vi "LockDelta_RH_v2.vi"() -> ()   [LabVIEW 2019]
uses:
  <vilib>/Analysis/baseanly.llb/Mean (DBL).vi
  DeltaRamp_globals.vi
  B_Globals.vi
  Global 2.vi
  <vilib>/Analysis/NI_AALBase.lvlib
panel:
  out "Remote_Save_String":string
  in  "L1 ID":string
  in  "D1 ID":string="52A"
  out "read buffer":string
  out "R2":dbl=1.74102008
  in  "D1_use":bool=TRUE
  in  "L1_use":bool
  in  "D1":refnum<visa-resource-name>="GPIB1::20::INSTR"
  in  "L1":refnum<visa-resource-name>="GPIB1::7::INSTR"
  in  "Freq":dbl=71.34 format="%#_6e"
  out "B_set [T]":dbl
  in  "Reading Delay [ms]":i32=20 min=5
  in  "RW Delay":i32=5
  out "Exec Time [ms]":u32=29
  in  "B/T":bool=TRUE
  in  "Smart Avs":bool=TRUE
  in  "Points":dbl=1.0
  out "PpP":dbl=8.0
  in  "Combo Box":string(combo)="Temp"
  in  "Save":bool
  in  "Abort Delta":bool
  out "B [T]":dbl
  in  "Arm":bool
  in  "Measure":bool
  in  "I_Max":dbl=5e-05
  out "T":cluster{"X":dbl[], "Y":dbl[]}[](graph)=[{"X"=[300.2348517520214, 300.17, 300.17799999999994, 300.1689999999999, 300.166, 300.18, 300.186, 300.212, 300.20699999999994, 300.192, 300.183, 300.174, 300.167, 300.181, 300.1689999999999, 300.147, 300.157, 300.163, 300.166, 300.172, 300.184, 300.176, 300.16, 300.152, 300.16, 300.145, 300.12899999999996, 300.153, 300.157, 300.164, 300.153, 300.158, 300.154, 300.16800000000006, 300.184, 300.18800000000005, 300.176, 300.17900000000003, 300.1480000000001, 300.14899999999994, 300.15900000000005, 300.15799999999996, 300.147, 300.138, 300.135, 300.1360000000001, 300.162, 300.152, 300.146, 300.162, 300.167, 300.175, 300.16800000000006, 300.173, 300.189, 300.194, 300.183, 300.19700000000006, 300.19, 300.183, 300.15900000000005, 300.126, 300.12899999999996, 300.13900000000007, 300.12899999999996, 300.099, 300.048, 300.029, 299.998, 299.936, 299.74499999999995, 299.46599999999995, 299.114, 298.872, 298.507, 298.157, 297.859, 297.579, 297.412, 297.182, 297.0059999999999, 296.854, 296.76400000000007, 296.657, 296.56300000000005, 296.491, 296.433, 296.375, 296.334, 296.319, 296.305, 296.27, 296.262, 296.25500000000005, 296.263, 296.27399999999994, 296.29300000000006, 296.32099999999997, 296.347, 296.383, 296.4189999999999, 296.449, 296.502, 296.57099999999997, 296.673, 296.728, 296.81, 296.886, 296.987, 297.075, 297.157, 297.282, 297.405, 297.542, 297.69700000000006, 297.782, 297.923, 298.048, 298.181, 298.263, 298.39899999999994, 298.537, 298.67, 298.799, 298.88900000000007, 299.002, 299.125, 299.252, 299.34, 299.45, 299.58199999999994, 299.709, 299.809, 299.872, 299.968, 300.061, 300.147, 300.23500000000007, 300.288, 300.36999999999995, 300.449, 300.511, 300.564, 300.59999999999997, 300.65900000000005, 300.7060000000001, 300.753, 300.796, 300.819, 300.839, 300.867, 300.887, 300.92900000000003, 300.951, 300.961, 300.98500000000007, 300.992, 301.00399999999996, 301.01400000000007, 301.01, 301.019, 301.017, 301.012, 301.00399999999996, 300.991, 300.969, 300.959, 300.9560000000001, 300.954, 300.93, 300.925, 300.921, 300.913, 300.904, 300.88900000000007, 300.855, 300.846, 300.833, 300.825, 300.786, 300.788], "Y"=[nan, nan, nan, nan, nan, nan, nan, nan, nan, nan, nan, nan, nan, nan, nan, nan, nan, nan, nan, nan, nan, nan, nan, nan, nan, nan, nan, nan, nan, nan, nan, nan, nan, nan, nan, nan, nan, nan, nan, nan, nan, nan, nan, nan, nan, nan, nan, nan, nan, nan, nan, nan, nan, nan, nan, nan, nan, nan, nan, nan, nan, nan, nan, nan, nan, nan, nan, nan, nan, nan, nan, nan, nan, nan, nan, nan, nan, nan, nan, nan, nan, nan, nan, nan, nan, nan, nan, nan, nan, nan, nan, nan, nan, nan, nan, nan, nan, nan, nan, nan, nan, nan, nan, nan, nan, nan, nan, nan, nan, nan, nan, nan, nan, nan, nan, nan, nan, nan, nan, nan, nan, nan, nan, nan, nan, nan, nan, nan, nan, nan, nan, nan, nan, nan, nan, nan, nan, nan, nan, nan, nan, nan, nan, nan, nan, nan, nan, nan, nan, nan, nan, nan, nan, nan, nan, nan, nan, nan, nan, nan, nan, nan, nan, nan, nan, nan, nan, nan, nan, nan, nan, nan, nan, nan, nan, nan, nan, nan, nan, nan, nan]}, {"X"=[300.2348517520214, 300.17, 300.17799999999994, 300.1689999999999, 300.166, 300.18, 300.186, 300.212, 300.20699999999994, 300.192, 300.183, 300.174, 300.167, 300.181, 300.1689999999999, 300.147, 300.157, 300.163, 300.166, 300.172, 300.184, 300.176, 300.16, 300.152, 300.16, 300.145, 300.12899999999996, 300.153, 300.157, 300.164, 300.153, 300.158, 300.154, 300.16800000000006, 300.184, 300.18800000000005, 300.176, 300.17900000000003, 300.1480000000001, 300.14899999999994, 300.15900000000005, 300.15799999999996, 300.147, 300.138, 300.135, 300.1360000000001, 300.162, 300.152, 300.146, 300.162, 300.167, 300.175, 300.16800000000006, 300.173, 300.189, 300.194, 300.183, 300.19700000000006, 300.19, 300.183, 300.15900000000005, 300.126, 300.12899999999996, 300.13900000000007, 300.12899999999996, 300.099, 300.048, 300.029, 299.998, 299.936, 299.74499999999995, 299.46599999999995, 299.114, 298.872, 298.507, 298.157, 297.859, 297.579, 297.412, 297.182, 297.0059999999999, 296.854, 296.76400000000007, 296.657, 296.56300000000005, 296.491, 296.433, 296.375, 296.334, 296.319, 296.305, 296.27, 296.262, 296.25500000000005, 296.263, 296.27399999999994, 296.29300000000006, 296.32099999999997, 296.347, 296.383, 296.4189999999999, 296.449, 296.502, 296.57099999999997, 296.673, 296.728, 296.81, 296.886, 296.987, 297.075, 297.157, 297.282, 297.405, 297.542, 297.69700000000006, 297.782, 297.923, 298.048, 298.181, 298.263, 298.39899999999994, 298.537, 298.67, 298.799, 298.88900000000007, 299.002, 299.125, 299.252, 299.34, 299.45, 299.58199999999994, 299.709, 299.809, 299.872, 299.968, 300.061, 300.147, 300.23500000000007, 300.288, 300.36999999999995, 300.449, 300.511, 300.564, 300.59999999999997, 300.65900000000005, 300.7060000000001, 300.753, 300.796, 300.819, 300.839, 300.867, 300.887, 300.92900000000003, 300.951, 300.961, 300.98500000000007, 300.992, 301.00399999999996, 301.01400000000007, 301.01, 301.019, 301.017, 301.012, 301.00399999999996, 300.991, 300.969, 300.959, 300.9560000000001, 300.954, 300.93, 300.925, 300.921, 300.913, 300.904, 300.88900000000007, 300.855, 300.846, 300.833, 300.825, 300.786, 300.788], "Y"=[1.7447801286792448, 1.7447222037500003, 1.7444892225, 1.7447247049999999, 1.7444935777777777, 1.7447010424999998, 1.7444126299999998, 1.7446228562500001, 1.7444523166666668, 1.7446782055555554, 1.7442503550000001, 1.7445815471428572, 1.7445446699999998, 1.7444733666666667, 1.74438583625, 1.74470474, 1.74432511625, 1.7444609047058823, 1.7444559175000003, 1.74453283875, 1.74436205, 1.74448020875, 1.74424474, 1.74459511, 1.7443100344444444, 1.7445789274999999, 1.7443861512499996, 1.7446031822222219, 1.7441049224999998, 1.74444188, 1.74417156, 1.7444447835294117, 1.74440267625, 1.7443347725000002, 1.74462658125, 1.7443272925, 1.7443892799999998, 1.7444658800000001, 1.74426717875, 1.7445588900000002, 1.7442914700000003, 1.7443815285714288, 1.7442203222222221, 1.7444356812500001, 1.7443279187500003, 1.7443443888235295, 1.7443939437500002, 1.74418871125, 1.744245395, 1.74435906125, 1.7442560699999998, 1.744363755, 1.7442435012500002, 1.7443550225000002, 1.744275161111111, 1.7444952322222225, 1.7442897475000003, 1.7442084155555557, 1.74446526125, 1.744032623333333, 1.7444503137499998, 1.74405478, 1.7443459487499997, 1.7442460844444443, 1.7442503712500002, 1.74424321875, 1.7442301224999996, 1.7443053200000003, 1.7443908711111114, 1.7441522625, 1.7443821125, 1.7443603274999997, 1.74452349625, 1.7445079087499997, 1.7445287322222223, 1.74465774, 1.7443728855555556, 1.7443117199999998, 1.744500492222222, 1.7439781575, 1.74443067625, 1.7438763237500001, 1.7443025377777777, 1.7439469600000002, 1.7432400377777781, 1.74333129625, 1.7434138362499998, 1.7431936575000002, 1.7430730922222224, 1.7426461137499998, 1.7430441525, 1.7426726075, 1.7428233350000002, 1.74276167125, 1.74255301125, 1.74272678625, 1.7424671522222224, 1.74262526625, 1.74249634125, 1.7425897587499999, 1.742324008888889, 1.7426337, 1.7422789637499998, 1.7422661775, 1.742301568888889, 1.74232783875, 1.74205565625, 1.7423048024999999, 1.7421523744444443, 1.741956101111111, 1.7423072912499997, 1.74186632, 1.7423694011111113, 1.7417824999999998, 1.7421789288888891, 1.7418095787499999, 1.74209737875, 1.74203477625, 1.7418068633333332, 1.74197279, 1.74173145, 1.7420101762500002, 1.7416327388888888, 1.7419502722222222, 1.74192201875, 1.74173143625, 1.7418395262500002, 1.7417157888888888, 1.74199148875, 1.74175852625, 1.74190086125, 1.7415953755555555, 1.742182105, 1.7419347633333333, 1.74175076125, 1.741818508888889, 1.74180181375, 1.74189556875, 1.7418619544444445, 1.7418426124999997, 1.7420506762499999, 1.7416219577777778, 1.7419721533333334, 1.7416080975, 1.7417956928571425, 1.7416463144444445, 1.7418566212500002, 1.7418234744444443, 1.7418127074999998, 1.742116705, 1.7417476175000002, 1.7418373433333332, 1.74178592875, 1.7417111975, 1.7420812188888888, 1.7416140275, 1.742021707777778, 1.741713985, 1.74195474375, 1.7416716374999999, 1.7419106966666666, 1.741797445, 1.741861925, 1.7417786377777775, 1.7419472487500003, 1.7416695899999999, 1.74205845625, 1.7417355025, 1.742054368888889, 1.74172237625, 1.74197687, 1.7418625233333334, 1.74192047125, 1.7420078655555553, 1.74175012125, 1.7421686799999998, 1.74217179375, 1.74163177625, 1.741930425, 1.7418367466666664, 1.7420905387499999]}] caption="XY Graph"
  in  "Reset":bool
  out "Spl T [K]":dbl=300.783
  out "R1 [Ohm]":dbl=nan
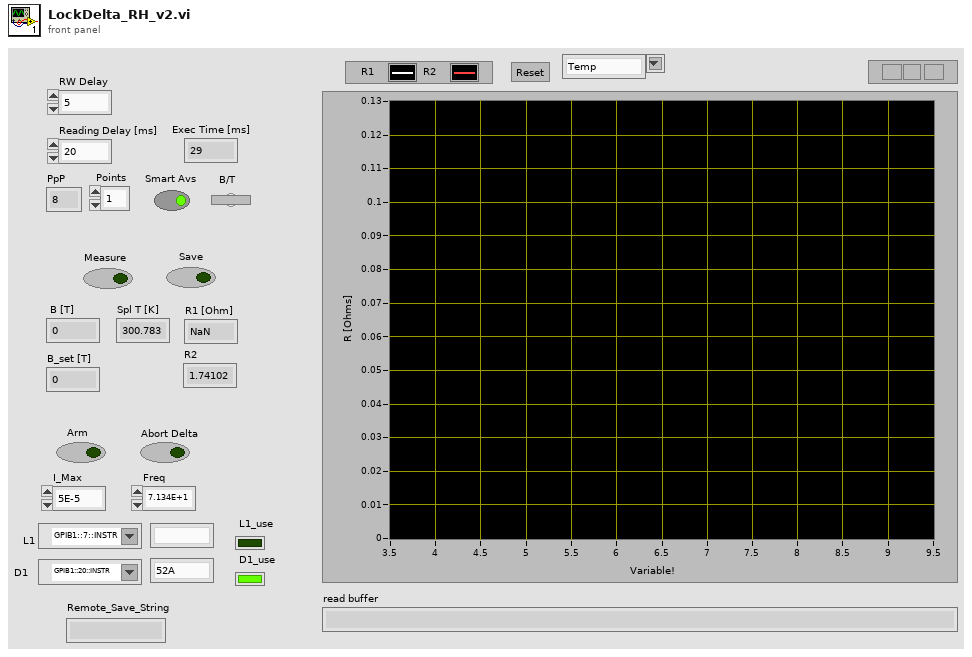
[diagram p1: front panel]
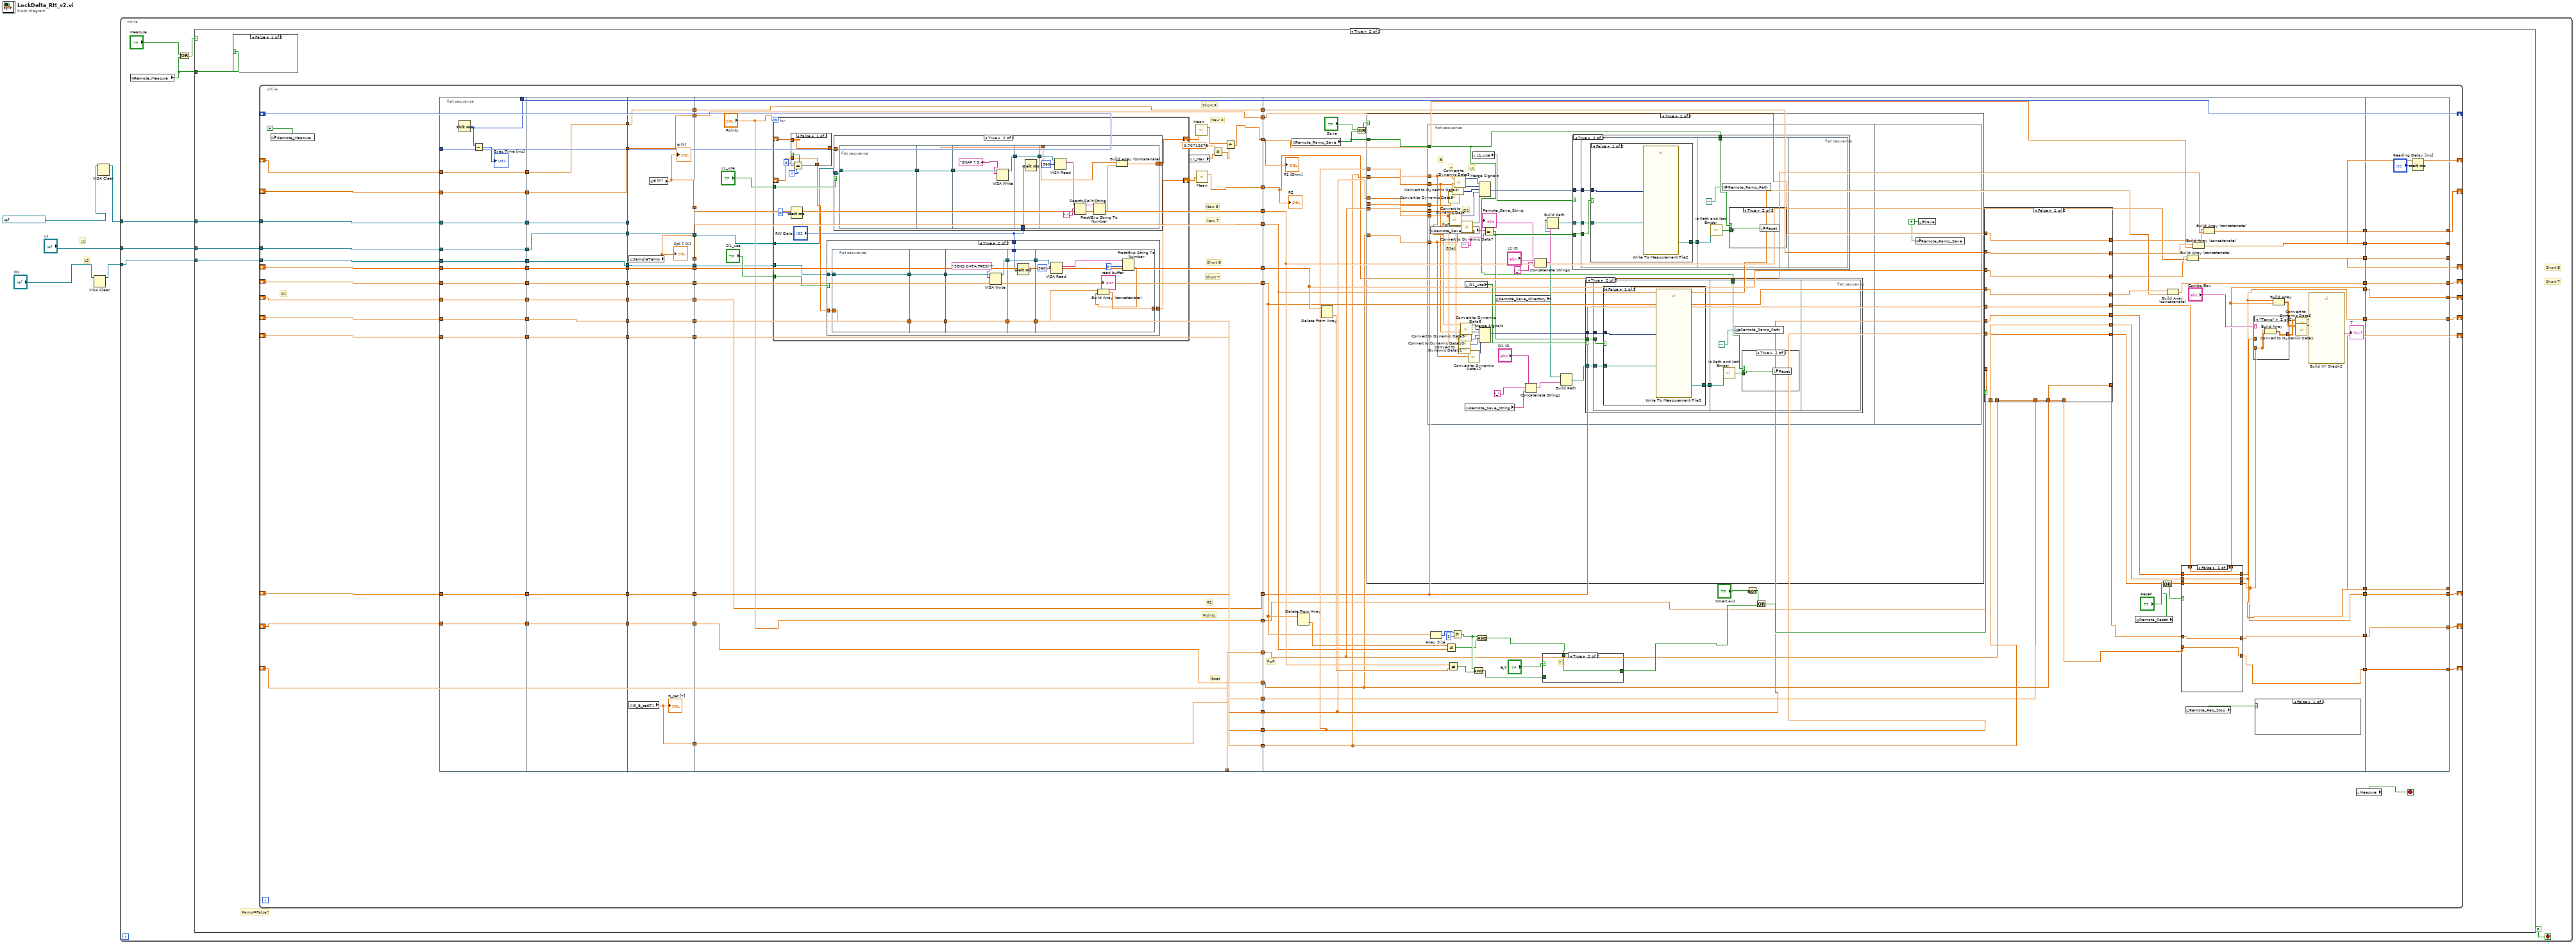
[diagram p0: block diagram]
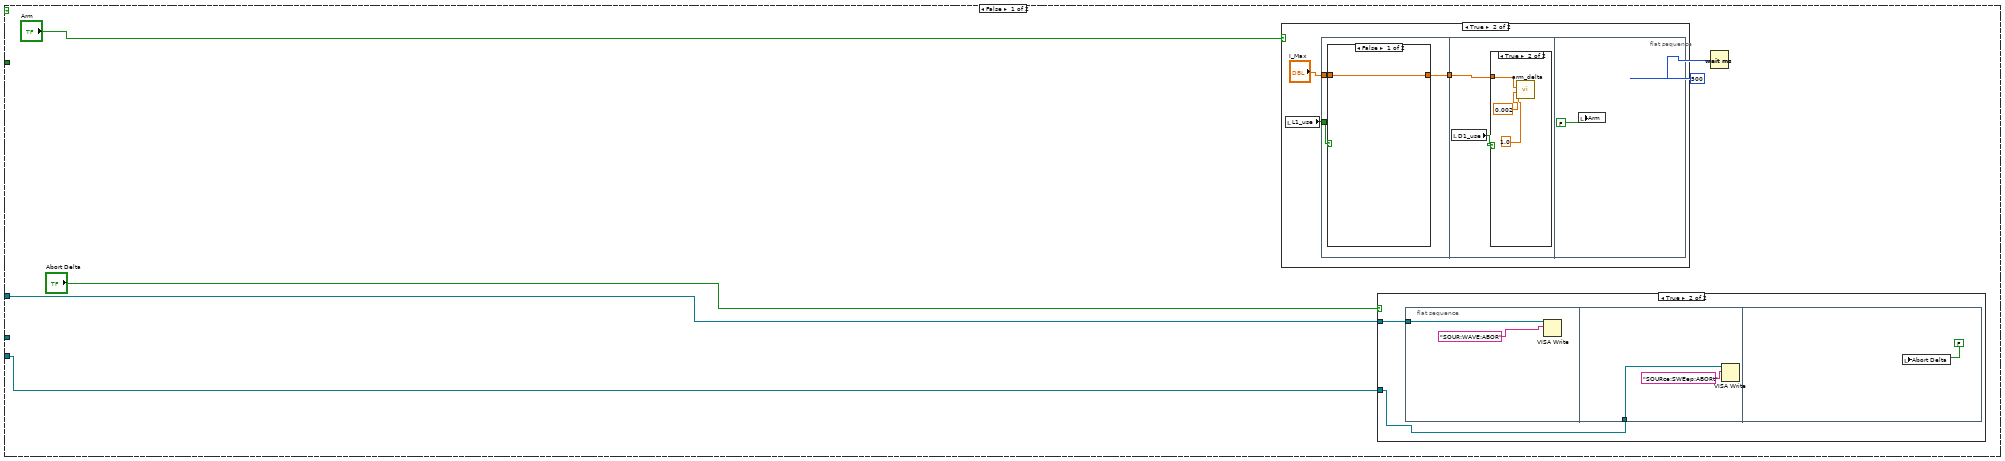
[diagram p2: hidden frame]
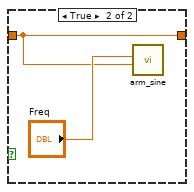
[diagram p5: hidden frame]
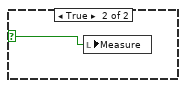
[diagram p7: hidden frame]
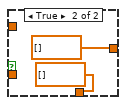
[diagram p10: hidden frame]
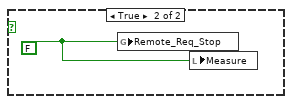
[diagram p12: hidden frame]
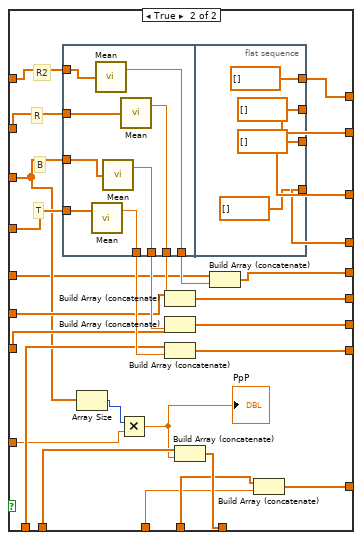
[diagram p13: hidden frame]
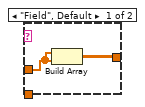
[diagram p14: hidden frame]
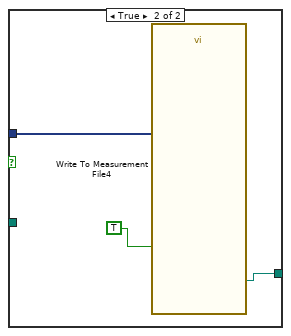
[diagram p17: hidden frame]
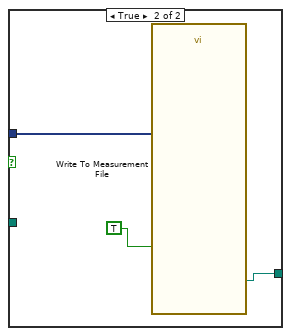
[diagram p20: hidden frame]
diagram:
  # "L2"
  # "L1"
  n1 = VISA Clear(VISA resource name="D1") -> (VISA resource name out=w1:refnum<visa-resource-name>)  [unwired: 1 in, 1 out]
  n2 = VISA Clear(VISA resource name=refnum<visa-resource-name> "GPIB1::22::INSTR" ("Keithley")) -> (VISA resource name out=w5:refnum<visa-resource-name>)  [unwired: 1 in, 1 out]
  n3 = while {
    tunnel: w5 -> [w11]
    tunnel: "L1" -> [w7]
    tunnel: w1 -> [w6]
    stop <- FALSE stop-if-true
    # "Short T"
    # "Short B"
    n4 = global read "DeltaRamp_globals.vi" "Remote_Measure"() -> (w8:bool)
    n5 = Or(x="Measure", y=w8) -> (x .or. y?=w10:bool)
    n6 = case shown="True" w10 {
      tunnel: w11 -> [w15 w43]
      tunnel: w8 -> [_ w42]
      tunnel: w7 -> [_ w41]
      tunnel: w6 -> [w13 w40]
      frame False {
        n7 = case shown="True" "Arm" {
          frame False {
          }
          frame True {
            n8 = local read "L1_use"() -> (w25:bool)
            n9 = flat-sequence {
              tunnel: [w30] -> w27
              tunnel: "I_Max" -> [w29]
              tunnel: w25 -> [w28]
              tunnel: w27 -> [w35]
              frame #0 {
                n10 = case shown="False" w28 {
                  tunnel: [w31 w32] -> w30
                  tunnel: w29 -> [w31 w32]
                  frame False {
                  }
                  frame True {
                    n11 = call "arm_sine.vi"("Peak Amp"=w32, "Freq"="Freq") -> ()  [unwired: 10 in]
                  }
                }
              }
              frame #1 {
                n12 = local read "D1_use"() -> (w34:bool)
                n13 = case shown="True" w34 {
                  tunnel: w35 -> [_ w38]
                  frame False {
                  }
                  frame True {
                    n14 = call "arm_delta.vi"("Compliance [V]"=1.0, "DELAY [sec]"=0.002, "I-HIGH [A]"=w38) -> ()  [unwired: 9 in]
                  }
                }
              }
              frame #2 {
                n15 = local write "Arm"(FALSE) -> ()
              }
            }
          }
        }
        n16 = case shown="True" "Abort Delta" {
          tunnel: w15 -> [_ w19]
          tunnel: w13 -> [_ w18]
          frame False {
          }
          frame True {
            n17 = flat-sequence {
              tunnel: w19 -> [w21]
              tunnel: w18 -> [w22]
              frame #0 {
                n18 = VISA Write(VISA resource name=w21, write buffer="SOUR:WAVE:ABOR") -> ()  [unwired: 1 in, 3 out]
              }
              frame #1 {
                n19 = VISA Write(VISA resource name=w22, write buffer="SOURce:SWEep:ABORt") -> ()  [unwired: 1 in, 3 out]
              }
              frame #2 {
                n20 = local write "Abort Delta"(FALSE) -> ()
              }
            }
          }
        }
        n21 = Wait (ms)(milliseconds to wait=500) -> ()  [unwired: 1 out]
      }
      frame True {
        # "Ramp=False?"
        n22 = case shown="False" w42 {
          selector: w42 -> [_ w44]
          frame False {
          }
          frame True {
            n23 = local write "Measure"(w44) -> ()
          }
        }
        n24 = while {
          shift-right: [w87] -> _
          shift-left: _ -> [w94]
          shift-right: [w106] -> _
          shift-left: _ -> [w111]
          tunnel: w43 -> [w129]
          shift-right: [w104] -> _
          shift-left: _ -> [w117]
          shift-right: [w86] -> _
          shift-left: _ -> [w98]
          shift-right: [w88] -> _
          shift-left: _ -> [w103]
          shift-right: [w105] -> _
          shift-left: _ -> [w121]
          shift-right: [w130] -> _
          shift-left: _ -> [w131]
          shift-right: [w133] -> _
          shift-left: _ -> [w134]
          shift-right: [w70] -> _
          shift-left: _ -> [w75]
          tunnel: w41 -> [w67]
          tunnel: w40 -> [w66]
          shift-right: [w52] -> _
          shift-left: _ -> [w57]
          shift-right: [w50] -> _
          shift-left: _ -> [w48]
          stop <- w77 stop-if-true
          # "R2"
          n25 = global write "DeltaRamp_globals.vi" "Remote_Measure"(FALSE) -> ()
          n26 = flat-sequence {
            tunnel: w134 -> [w150]
            tunnel: [w148] -> w133
            tunnel: w129 -> [w147]
            tunnel: [w147] -> w127
            tunnel: w121 -> [w146]
            tunnel: [w146] -> w120
            tunnel: w117 -> [w145]
            tunnel: [w145] -> w114
            tunnel: w111 -> [w144]
            tunnel: [w144] -> w109
            tunnel: w103 -> [w143]
            tunnel: [w143] -> w100
            tunnel: [w142] -> w99
            tunnel: w98 -> [w142]
            tunnel: [w141] -> w95
            tunnel: w94 -> [w141]
            tunnel: [w140] -> w76
            tunnel: w75 -> [w140]
            tunnel: w67 -> [w139]
            tunnel: w66 -> [w138]
            tunnel: [w139] -> w65
            tunnel: [w138] -> w64
            tunnel: [w137] -> w58
            tunnel: w57 -> [w137]
            tunnel: [w136] -> w49
            tunnel: w48 -> [w136]
            tunnel: [w162] -> w128
            tunnel: w127 -> [w162]
            tunnel: w120 -> [w161]
            tunnel: [w161] -> w119
            tunnel: [w160] -> w115
            tunnel: w114 -> [w160]
            tunnel: [w159] -> w110
            tunnel: w109 -> [w159]
            tunnel: [w158] -> w101
            tunnel: w100 -> [w158]
            tunnel: w99 -> [w157]
            tunnel: [w157] -> w96
            tunnel: w95 -> [w156]
            tunnel: [w156] -> w92
            tunnel: w76 -> [w155]
            tunnel: [w155] -> w73
            tunnel: w65 -> [w154]
            tunnel: w64 -> [w153]
            tunnel: [w154] -> w62
            tunnel: [w153] -> w60
            tunnel: w58 -> [w152]
            tunnel: [w152] -> w56
            tunnel: w49 -> [w151]
            tunnel: [w151] -> w46
            tunnel: w128 -> [_]
            tunnel: [w176] -> w125
            tunnel: [w175] -> w123
            tunnel: w119 -> [w174]
            tunnel: [w174] -> w118
            tunnel: [w173] -> w116
            tunnel: w115 -> [w173]
            tunnel: w110 -> [w172]
            tunnel: [w172] -> w108
            tunnel: [w171] -> w102
            tunnel: w101 -> [w171]
            tunnel: [w170] -> w97
            tunnel: w96 -> [w170]
            tunnel: [w169] -> w93
            tunnel: w92 -> [w169]
            tunnel: [w168] -> w74
            tunnel: w73 -> [w168]
            tunnel: [w167] -> w69
            tunnel: [w166] -> w63
            tunnel: w62 -> [w166]
            tunnel: [w165] -> w61
            tunnel: w60 -> [w165]
            tunnel: w56 -> [w164]
            tunnel: [w164] -> w54
            tunnel: [w163] -> w47
            tunnel: w46 -> [w163]
            tunnel: [w201] -> w132
            tunnel: w131 -> [w201]
            tunnel: [w181] -> w126
            tunnel: w125 -> [w200]
            tunnel: [w200] -> w124
            tunnel: w123 -> [w199]
            tunnel: [w199] -> w122
            tunnel: w118 -> [w198]
            tunnel: w116 -> [w197]
            tunnel: [w198] -> w113
            tunnel: [w197] -> w112
            tunnel: w108 -> [w196]
            tunnel: [w196] -> w107
            tunnel: w102 -> [w195]
            tunnel: w97 -> [w194]
            tunnel: w93 -> [w193]
            tunnel: [w195] -> w91
            tunnel: [w194] -> w90
            tunnel: [w193] -> w89
            tunnel: ["Points"] -> w85
            tunnel: w74 -> [w191]
            tunnel: [w191] -> w72
            tunnel: w69 -> [w190]
            tunnel: [w190] -> w68
            tunnel: w63 -> [w186]
            tunnel: w61 -> [w187]
            tunnel: [w177] -> w59
            tunnel: [w183] -> w55
            tunnel: w54 -> [w183]
            tunnel: w47 -> [w182]
            tunnel: [w182] -> w45
            tunnel: w132 -> [w313]
            tunnel: w126 -> [w305]
            tunnel: w124 -> [w304]
            tunnel: w122 -> [w300]
            tunnel: w113 -> [w309]
            tunnel: w112 -> [w303]
            tunnel: w107 -> [w308]
            tunnel: w91 -> [w292]
            tunnel: w90 -> [w291]
            tunnel: w89 -> [w290]
            tunnel: w85 -> [w296]
            tunnel: [w297] -> w84
            tunnel: [w306] -> w83
            tunnel: [w302] -> w82
            tunnel: [w301] -> w81
            tunnel: [w279] -> w80
            tunnel: [w299] -> w79
            tunnel: [w298] -> w78
            tunnel: w72 -> [w293]
            tunnel: [w295] -> w71
            tunnel: w68 -> [w289]
            tunnel: w59 -> [w285]
            tunnel: w55 -> [w288]
            tunnel: [w286] -> w53
            tunnel: [w281] -> w51
            tunnel: w45 -> [w283]
            tunnel: [w504] -> w86
            tunnel: [w505] -> w87
            tunnel: [w506] -> w88
            tunnel: [w507] -> w104
            tunnel: [w508] -> w105
            tunnel: [w509] -> w106
            tunnel: [w510] -> w130
            tunnel: w84 -> [w510]
            tunnel: w83 -> [w509]
            tunnel: w82 -> [w508]
            tunnel: w81 -> [w507]
            tunnel: w80 -> [w506]
            tunnel: w79 -> [w505]
            tunnel: w78 -> [w504]
            tunnel: w71 -> [w502]
            tunnel: [w502] -> w70
            tunnel: [w501] -> w52
            tunnel: w53 -> [w501]
            tunnel: w51 -> [w500]
            tunnel: [w500] -> w50
            frame #0 {
              n27 = Tick Count (ms)() -> (millisecond timer value=w148:u32)
              n28 = Subtract(x=w148, y=w150) -> (x-y=→"Exec Time [ms]":u32)
            }
            frame #1 {
            }
            frame #2 {
              n29 = global read "Global 2.vi" "SampleTemp"() -> (w175:dbl)
              "Spl T [K]" <- w175
              n30 = global read "B_Globals.vi" "G_B_set[T]"() -> (w167:dbl)
              "B_set [T]" <- w167
              n31 = global read "B_Globals.vi" "B [T]"() -> (w176:dbl)
              "B [T]" <- w176
            }
            frame #3 {
              # "R2"
              # "Bset"
              # "Points"
              # "Short R"
              # "New T"
              # "New B"
              # "Short T"
              # "Short B"
              # "New R"
              n32 = for {
                N: "Points" -> [_]
                shift-right: [w208] -> w202
                shift-left: _ -> [w214]
                tunnel: "D1_use" -> [w213]
                tunnel: "L1_use" -> [w212]
                tunnel: w187 -> [w211]
                tunnel: w186 -> [w210]
                shift-right: [w205] -> w185
                shift-left: _ -> [w207]
                i -> [w215]
                n33 = Wait (ms)(milliseconds to wait=0) -> ()  [unwired: 1 out]
                n34 = Equal?(x=0, y=w215) -> (x = y?=w217:bool)
                n35 = case shown="False" w217 {
                  tunnel: [w274 dbl[] [] ("Numeric")] -> w209
                  tunnel: w214 -> [w274 _]
                  tunnel: w207 -> [w273 _]
                  tunnel: [w273 dbl[] [] ("Numeric")] -> w206
                  frame False {
                  }
                  frame True {
                  }
                }
                n36 = case shown="True" w213 {
                  tunnel: w211 -> [_ w250]
                  tunnel: w206 -> [w242 w249]
                  tunnel: [w242 w244] -> w205
                  tunnel: "RW Delay" -> [_ w243]
                  frame False {
                  }
                  frame True {
                    n37 = flat-sequence {
                      tunnel: w250 -> [w256]
                      tunnel: [w256] -> w254
                      tunnel: w249 -> [w255]
                      tunnel: [w255] -> w247
                      tunnel: w254 -> [w258]
                      tunnel: [w258] -> w253
                      tunnel: [w257] -> w248
                      tunnel: w247 -> [w257]
                      tunnel: [w261] -> w252
                      tunnel: w253 -> [w262]
                      tunnel: w248 -> [w259]
                      tunnel: [w259] -> w245
                      tunnel: [w265] -> w251
                      tunnel: w252 -> [w265]
                      tunnel: [w264] -> w246
                      tunnel: w245 -> [w264]
                      tunnel: w243 -> [w263]
                      tunnel: w251 -> [w271]
                      tunnel: w246 -> [w270]
                      tunnel: [w269] -> w244
                      frame #0 {
                      }
                      frame #1 {
                      }
                      frame #2 {
                        n38 = VISA Write(VISA resource name=w262, write buffer="SENS:DATA:FRESh?") -> (VISA resource name out=w261:refnum<visa-resource-name>)  [unwired: 1 in, 2 out]
                      }
                      frame #3 {
                        n39 = Wait (ms)(milliseconds to wait=w263) -> ()  [unwired: 1 out]
                      }
                      frame #4 {
                        n40 = VISA Read(VISA resource name=w271, byte count=u32 360) -> (read buffer=w267:string)  [unwired: 1 in, 3 out]
                        n41 = Fract/Exp String To Number(string=w267, offset=0) -> (number=w266:dbl)  [unwired: 3 out]
                        n42 = Build Array (concatenate)(w270, w266) -> (w269:dbl[])
                      }
                    }
                  }
                }
                n43 = case shown="True" w212 {
                  tunnel: w210 -> [_ w222]
                  tunnel: w209 -> [w218 w221]
                  tunnel: [w218 w220] -> w208
                  tunnel: "RW Delay" -> [_ w219]
                  frame False {
                  }
                  frame True {
                    n44 = flat-sequence {
                      tunnel: w222 -> [w227]
                      tunnel: [w227] -> w226
                      tunnel: w226 -> [w228]
                      tunnel: [w228] -> w225
                      tunnel: [w230] -> w224
                      tunnel: w225 -> [w231]
                      tunnel: [w233] -> w223
                      tunnel: w224 -> [w233]
                      tunnel: w219 -> [w232]
                      tunnel: w223 -> [w240]
                      tunnel: w221 -> [w239]
                      tunnel: [w238] -> w220
                      frame #0 {
                      }
                      frame #1 {
                      }
                      frame #2 {
                        n45 = VISA Write(VISA resource name=w231, write buffer="SNAP ? 3,4") -> (VISA resource name out=w230:refnum<visa-resource-name>)  [unwired: 1 in, 2 out]
                      }
                      frame #3 {
                        n46 = Wait (ms)(milliseconds to wait=w232) -> ()  [unwired: 1 out]
                      }
                      frame #4 {
                        n47 = VISA Read(VISA resource name=w240, byte count=u32 360) -> (read buffer=w236:string)  [unwired: 1 in, 3 out]
                        n48 = Search/Split String(string=w236, search string/char (-)=",") -> (substring before match=w235:string)  [unwired: 1 in, 2 out]
                        n49 = Fract/Exp String To Number(string=w235) -> (number=w234:dbl)  [unwired: 1 in, 3 out]
                        n50 = Build Array (concatenate)(w239, w234) -> (w238:dbl[])
                      }
                    }
                  }
                }
              }
              n51 = local read "I_Max"() -> (w179:dbl)
              n52 = call-poly <vilib>:"Mean.vi"("X"=w202) -> ("mean"=w184:dbl)  [unwired: 1 out]
              n53 = call-poly <vilib>:"Mean.vi"("X"=w185) -> ("mean"=w177:dbl)  [unwired: 1 out]
              n54 = Multiply(x=0.70710678, y=w179) -> (x*y=w180:dbl)
              n55 = Divide(x=w184, y=w180) -> (x/y=w181:dbl)
            }
            frame #4 {
              # "PpP"
              n56 = global read "DeltaRamp_globals.vi" "Remote_Ramp_Save"() -> (w325:bool)
              n57 = Delete From Array(array=w303) -> (deleted portion=w311:dbl)  [unwired: 2 in, 1 out]
              n58 = Delete From Array(array=w309) -> (deleted portion=w310:dbl)  [unwired: 2 in, 1 out]
              n59 = Or(x="Save", y=w325) -> (x .or. y?=w320:bool)
              n60 = case shown="True" w320 {
                tunnel: w325 -> [_ w403]
                tunnel: w313 -> [_ w402]
                tunnel: w293 -> [_ w398]
                tunnel: w292 -> [_ w401]
                tunnel: w291 -> [_ w400]
                tunnel: w290 -> [_ w399]
                tunnel: w283 -> [_ w397]
                frame False {
                }
                frame True {
                  n61 = flat-sequence {
                    tunnel: w403 -> [w416]
                    tunnel: w402 -> [w423]
                    tunnel: w401 -> [w436]
                    tunnel: w400 -> [w429]
                    tunnel: w399 -> [w427]
                    tunnel: w398 -> [w421]
                    tunnel: w397 -> [w425]
                    frame #0 {
                      # "BSet"
                      # "PpP"
                      # "D1"
                      # "L1"
                      # "T"
                      # "B"
                      n62 = global read "DeltaRamp_globals.vi" "Remote_Save_String"() -> (w405:string)
                      "Remote_Save_String" <- w405
                      n63 = call "Convert to Dynamic Data5"("Array"=w436) -> ("Dynamic Data Type"=w433:dynamicdata)  [unwired: 3 in]
                      n64 = call "Convert to Dynamic Data"("Array"=w423) -> ("Dynamic Data Type"=w432:dynamicdata)  [unwired: 3 in]
                      n65 = call "Convert to Dynamic Data4"("Array"=w427) -> ("Dynamic Data Type"=w434:dynamicdata)  [unwired: 3 in]
                      n66 = call "Convert to Dynamic Data3"("Array"=w429) -> ("Dynamic Data Type"=w435:dynamicdata)  [unwired: 3 in]
                      n67 = call "Convert to Dynamic Data10"("Array"=w425) -> ("Dynamic Data Type"=w424:dynamicdata)  [unwired: 3 in]
                      n68 = call "Convert to Dynamic Data11"("Array"=w423) -> ("Dynamic Data Type"=w422:dynamicdata)  [unwired: 3 in]
                      n69 = call "Convert to Dynamic Data9"("Array"=w427) -> ("Dynamic Data Type"=w426:dynamicdata)  [unwired: 3 in]
                      n70 = call "Convert to Dynamic Data8"("Array"=w429) -> ("Dynamic Data Type"=w428:dynamicdata)  [unwired: 3 in]
                      n71 = call "Convert to Dynamic Data7"("Array"=w421) -> ("Dynamic Data Type"=w431:dynamicdata)  [unwired: 3 in]
                      n72 = local read "D1_use"() -> (w417:bool)
                      n73 = global read "DeltaRamp_globals.vi" "Remote_Save_String"() -> (w407:string)
                      n74 = call "Convert to Dynamic Data12"("Array"=w421) -> ("Dynamic Data Type"=w420:dynamicdata)  [unwired: 3 in]
                      n75 = local read "L1_use"() -> (w418:bool)
                      n76 = Merge Signals(w435, w434, w433, w432, w431) -> (w437:dynamicdata)
                      n77 = Merge Signals(w428, w426, w424, w422, w420) -> (w430:dynamicdata)
                      n78 = Equal?(x=w405, y="") -> (x = y?=w419:bool)
                      n79 = global read "DeltaRamp_globals.vi" "Remote_Save_Directory"() -> (w411:path)
                      n80 = Concatenate Strings("D1 ID", "_", w407) -> (w409:string)
                      n81 = Concatenate Strings("L1 ID", "_", w405) -> (w413:string)
                      n82 = Build Path(base path=w411, name or relative path=w413) -> (appended path=w412:path)
                      n83 = Build Path(base path=w411, name or relative path=w409) -> (appended path=w408:path)
                      n84 = case shown="True" w418 {
                        tunnel: w437 -> [_ w461]
                        tunnel: w419 -> [_ w460]
                        tunnel: w416 -> [_ w459]
                        tunnel: w412 -> [_ w458]
                        frame False {
                        }
                        frame True {
                          n85 = flat-sequence {
                            tunnel: w461 -> [w466]
                            tunnel: w460 -> [w465]
                            tunnel: [w464] -> w462
                            tunnel: w458 -> [w463]
                            tunnel: w462 -> [w475]
                            tunnel: w459 -> [w474]
                            frame #0 {
                              n86 = case shown="False" w465 {
                                tunnel: w466 -> [w469 w471]
                                tunnel: [w468 w470] -> w464
                                tunnel: w463 -> [w467 _]
                                frame False {
                                n87 = call "Write To Measurement File2"("Signals"=w469, "Filename"=w467) -> ("Filename Out"=w468:path)  [unwired: 15 in, 2 out]
                                }
                                frame True {
                                n88 = call "Write To Measurement File"("Signals"=w471, "Reset"=TRUE) -> ("Filename Out"=w470:path)  [unwired: 15 in, 2 out]
                                }
                              }
                            }
                            frame #1 {
                              n89 = call <vilib>:"Is Path and Not Empty.vi"("path"=w475) -> ("Is Path and Not Empty?"=w473:bool)  [unwired: 4 in]
                              n90 = global write "DeltaRamp_globals.vi" "Remote_Ramp_Path"(path "") -> ()
                              n91 = case shown="True" w474 {
                                tunnel: w473 -> [_ w477]
                                frame False {
                                }
                                frame True {
                                n92 = local write "Reset"(w477) -> ()
                                }
                              }
                            }
                            frame #2 {
                            }
                          }
                        }
                      }
                      n93 = case shown="True" w417 {
                        tunnel: w430 -> [_ w441]
                        tunnel: w408 -> [_ w440]
                        tunnel: w416 -> [_ w439]
                        tunnel: w419 -> [_ w438]
                        frame False {
                        }
                        frame True {
                          n94 = flat-sequence {
                            tunnel: w441 -> [w446]
                            tunnel: w440 -> [w445]
                            tunnel: [w444] -> w442
                            tunnel: w438 -> [w443]
                            tunnel: w442 -> [w455]
                            tunnel: w439 -> [w454]
                            frame #0 {
                              n95 = case shown="False" w443 {
                                tunnel: w446 -> [w449 w451]
                                tunnel: w445 -> [w448 _]
                                tunnel: [w447 w450] -> w444
                                frame False {
                                n96 = call "Write To Measurement File3"("Signals"=w449, "Filename"=w448) -> ("Filename Out"=w447:path)  [unwired: 15 in, 2 out]
                                }
                                frame True {
                                n97 = call "Write To Measurement File4"("Signals"=w451, "Reset"=TRUE) -> ("Filename Out"=w450:path)  [unwired: 15 in, 2 out]
                                }
                              }
                            }
                            frame #1 {
                              n98 = call <vilib>:"Is Path and Not Empty.vi"("path"=w455) -> ("Is Path and Not Empty?"=w453:bool)  [unwired: 4 in]
                              n99 = global write "DeltaRamp_globals.vi" "Remote_Ramp_Path"(path "") -> ()
                              n100 = case shown="True" w454 {
                                tunnel: w453 -> [_ w457]
                                frame False {
                                }
                                frame True {
                                n101 = local write "Reset"(w457) -> ()
                                }
                              }
                            }
                            frame #2 {
                            }
                          }
                        }
                      }
                    }
                    frame #1 {
                      w478 = FALSE
                      n102 = global write "DeltaRamp_globals.vi" "Remote_Ramp_Save"(w478) -> ()
                      n103 = local write "Save"(w478) -> ()
                    }
                  }
                }
              }
              n104 = Array Size(array=w303) -> (size(s)=w330:i32)
              n105 = Not Equal?(x=w311, y=w300) -> (x != y?=w331:bool)
              n106 = Not Equal?(x=w304, y=w310) -> (x != y?=w334:bool)
              n107 = Greater?(x=w330, y=1) -> (0:w333:bool)
              n108 = And(x=w333, y=w334) -> (x .and. y?=w335:bool)
              n109 = And(x=w333, y=w331) -> (x .and. y?=w336:bool)
              n110 = case shown="True" "B/T" {
                tunnel: w335 -> [w340 _]
                tunnel: w336 -> [_ w341]
                tunnel: [w340 w341] -> w337
                frame False {
                  # "B"
                }
                frame True {
                  # "T"
                }
              }
              n111 = Not(x="Smart Avs") -> (.not. x?=w327:bool)
              n112 = Or(x=w327, y=w337) -> (x .or. y?=w328:bool)
              n113 = case shown="False" w328 {
                tunnel: [w351 w380] -> w339
                tunnel: [w349 w379] -> w307
                tunnel: [w350 w366] -> w338
                tunnel: [w346 w377] -> w316
                tunnel: [w348 w376] -> w317
                tunnel: [w347 w374] -> w318
                tunnel: [w352 w372] -> w312
                tunnel: w313 -> [w352 w371]
                tunnel: w309 -> [w351 w362]
                tunnel: w303 -> [w350 w367]
                tunnel: w308 -> [w349 w368]
                tunnel: w292 -> [w348 w365]
                tunnel: w291 -> [w346 w364]
                tunnel: w290 -> [w347 w363]
                tunnel: w296 -> [_ w361]
                tunnel: w293 -> [w345 w360]
                tunnel: [w345 w359] -> w294
                tunnel: w289 -> [_ w358]
                tunnel: w288 -> [w344 w357]
                tunnel: [w344 w356] -> w287
                tunnel: [w343 w354] -> w284
                tunnel: w283 -> [w343 w353]
                frame False {
                }
                frame True {
                  # "R2"
                  # "T"
                  # "B"
                  # "R"
                  n114 = flat-sequence {
                    tunnel: [w387] -> w378
                    tunnel: [w386] -> w373
                    tunnel: [w388] -> w375
                    tunnel: w368 -> [w385]
                    tunnel: w362 -> [w384]
                    tunnel: w367 -> [w383]
                    tunnel: w357 -> [w382]
                    tunnel: [w381] -> w355
                    tunnel: [dbl[] []] -> w366
                    tunnel: [dbl[] []] -> w380
                    tunnel: [dbl[] []] -> w379
                    tunnel: [dbl[] []] -> w356
                    frame #0 {
                      n115 = call-poly <vilib>:"Mean.vi"("X"=w383) -> ("mean"=w388:dbl)  [unwired: 1 out]
                      n116 = call-poly <vilib>:"Mean.vi"("X"=w382) -> ("mean"=w381:dbl)  [unwired: 1 out]
                      n117 = call-poly <vilib>:"Mean.vi"("X"=w384) -> ("mean"=w387:dbl)  [unwired: 1 out]
                      n118 = call-poly <vilib>:"Mean.vi"("X"=w385) -> ("mean"=w386:dbl)  [unwired: 1 out]
                    }
                    frame #1 {
                    }
                  }
                  n119 = Array Size(array=w362) -> (size(s)=w370:i32)
                  n120 = Multiply(x=w370, y=w361) -> (x*y=w369:dbl)
                  "PpP" <- w369
                  n121 = Build Array (concatenate)(w365, w373) -> (w376:dbl[])
                  n122 = Build Array (concatenate)(w364, w378) -> (w377:dbl[])
                  n123 = Build Array (concatenate)(w363, w375) -> (w374:dbl[])
                  n124 = Build Array (concatenate)(w371, w369) -> (w372:dbl[])
                  n125 = Build Array (concatenate)(w353, w355) -> (w354:dbl[])
                  n126 = Build Array (concatenate)(w360, w358) -> (w359:dbl[])
                }
              }
              n127 = global read "DeltaRamp_globals.vi" "Remote_Reset"() -> (w321:bool)
              n128 = Or(x="Reset", y=w321) -> (x .or. y?=w323:bool)
              n129 = Build Array (concatenate)(w338, w300) -> (w301:dbl[])
              n130 = case shown="False" w323 {
                tunnel: w316 -> [w484 w493]
                tunnel: [w484 w492] -> w298
                tunnel: w318 -> [w483 w491]
                tunnel: [w483 w490] -> w299
                tunnel: [w482 w489] -> w279
                tunnel: w317 -> [w482 _]
                tunnel: [w481 w487] -> w297
                tunnel: w312 -> [w481 _]
                tunnel: [w480 w486] -> w295
                tunnel: w294 -> [w480 _]
                tunnel: w284 -> [w479 _]
                tunnel: [w479 w485] -> w281
                frame False {
                }
                frame True {
                  w488 = FALSE
                  n131 = flat-sequence {
                    tunnel: w493 -> [_]
                    tunnel: w491 -> [_]
                    tunnel: [dbl[] []] -> w490
                    tunnel: [dbl[] []] -> w492
                    tunnel: [dbl[] []] -> w489
                    tunnel: [dbl[] [] ("Numeric")] -> w487
                    tunnel: [dbl[] [] ("Numeric")] -> w486
                    tunnel: [dbl[] [] ("Numeric")] -> w485
                    frame #0 {
                    }
                  }
                  n132 = global write "DeltaRamp_globals.vi" "Remote_Reset"(w488) -> ()
                  n133 = local write "Reset"(w488) -> ()
                }
              }
              n134 = global read "DeltaRamp_globals.vi" "Remote_Req_Stop"() -> (w324:bool)
              n135 = Build Array (concatenate)(w339, w304) -> (w302:dbl[])
              n136 = Build Array (concatenate)(w307, w305) -> (w306:dbl[])
              n137 = Build Array (concatenate)(w287, w285) -> (w286:dbl[])
              n138 = case shown="\"Temp\"" "Combo Box" {
                tunnel: w299 -> [_ w396]
                tunnel: w298 -> [w394 _]
                tunnel: [w393 w395] -> w278
                frame "Field", Default {
                  n139 = Build Array(w394, w394) -> (w393:dbl[][])
                }
                frame "Temp" {
                  n140 = Build Array(w396, w396) -> (w395:dbl[][])
                }
              }
              n141 = case shown="False" w324 {
                frame False {
                }
                frame True {
                  w342 = FALSE
                  n142 = global write "DeltaRamp_globals.vi" "Remote_Req_Stop"(w342) -> ()
                  n143 = local write "Measure"(w342) -> ()
                }
              }
              n144 = Build Array(w279, w281) -> (w282:dbl[][])
              n145 = call "Convert to Dynamic Data6"("2D Array"=w278) -> ("Dynamic Data Type"=w277:dynamicdata)  [unwired: 3 in]
              n146 = call "Convert to Dynamic Data2"("2D Array"=w282) -> ("Dynamic Data Type"=w280:dynamicdata)  [unwired: 3 in]
              n147 = call "Build XY Graph2"("Y Input"=w280, "X Input"=w277) -> ("XY Graph"=→"T":cluster{"X":dbl[], "Y":dbl[]}[])  [unwired: 8 in, 1 out]
              "R1 [Ohm]" <- w305
              "R2" <- w285
            }
            frame #5 {
              n148 = Wait (ms)(milliseconds to wait="Reading Delay [ms]") -> ()  [unwired: 1 out]
            }
          }
          n149 = local read "Measure"() -> (w77:bool)
        }
      }
    }
  }
